vi "StartProcesses.vi"(8 "error in (no error)":errorcluster, 11 "SMO":refnum<class "SMO.lvclass">) -> (0 "error out":errorcluster, 3 "SMO out":refnum<class "SMO.lvclass">)   [LabVIEW 2013, in "SMO.lvclass"]
doc: "---------------------------------------------------------------\nJKI State Machine Objects™\nhttp://jki.net/state-machine-objects/\nCopyright (C) 2005-2015, JKI <info@jki.net>\nALL RIGHTS RESERVED"
uses:
  SMO.lvclass
panel:
  # "For instructions on how to use the JKI State Machine Objects, examples and video tutorials, visit:\nhttp://jki.net/state-machine-objects/\n\nJKI State Machine Objects™\nhttp://jki.net/state-machine-objects/\nCopyright (C) 2005-2015, JKI <info@jki.net>\nALL RIGHTS RESERVED"
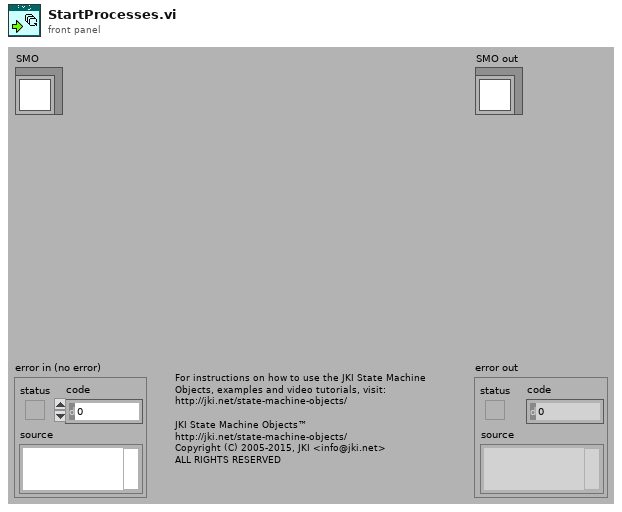
[diagram p1: front panel]
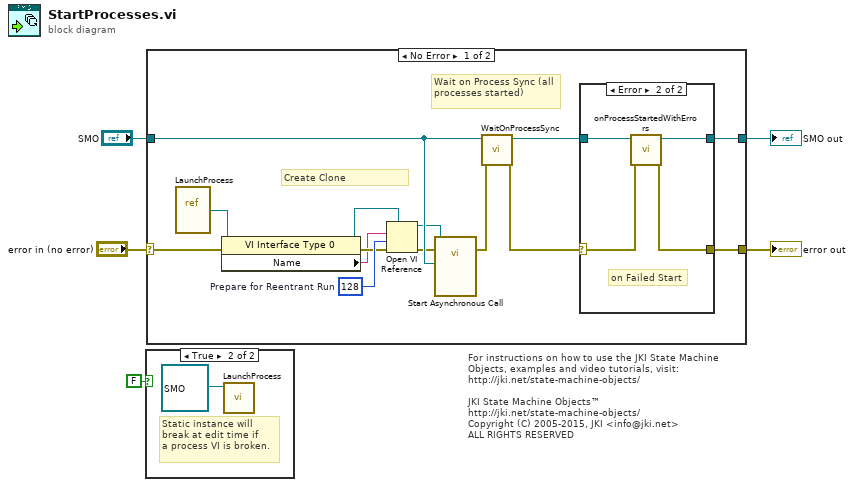
[diagram p0: block diagram]
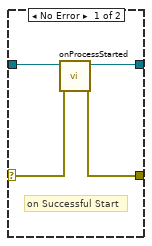
[diagram p3: hidden frame]
diagram:
  # "For instructions on how to use the JKI State Machine Objects, examples and video tutorials, visit:\nhttp://jki.net/state-machine-objects/\n\nJKI State Machine Objects™\nhttp://jki.net/state-machine-objects/\nCopyright (C) 2005-2015, JKI <info@jki.net>\nALL RIGHTS RESERVED"
  n1 = case shown="True" FALSE {
    frame False {
    }
    frame True {
      # "Static instance will\nbreak at edit time if\na process VI is broken."
      n2 = call "LaunchProcess.vi"("SMO Reference"=refnum<class "SMO.lvclass"> refnum ("JKI SMO.lvclass")) -> ()  [unwired: 11 in]
    }
  }
  n3 = case shown="No Error" "error in (no error)" {
    selector: "error in (no error)" -> [w20 w30]
    tunnel: [w17 w30] -> w2
    tunnel: "SMO" -> [w14 w29]
    tunnel: [w15 w29] -> w3
    frame No Error {
      w13 = 128  # Prepare for Reentrant Run
      # "Create Clone"
      # "Wait on Process Sync (all processes started)"
      n4 = vi-ref "LaunchProcess.vi"() -> (w9:refnum<vi>)
      n5 = property class="VI Interface Type 0"(reference=w9, error in=w20) -> (reference out=w10:refnum<vi>, error out=w12:errorcluster, "Name"=w11:string)
      n6 = Open VI Reference(type specifier VI Refnum (for type only)=w10, vi path=w11, options=w13, error in (no error)=w12) -> (vi reference=w7:refnum<vi>, error out=w8:errorcluster)  [unwired: 1 in, 1 out]
      n7 = call-by-ref "Start Asynchronous Call"(reference=w7, error in=w8, "SMO Reference"=w14) -> (error out=w19:errorcluster)  [unwired: 11 in, 1 out]
      n8 = call "WaitOnProcessSync.vi"("error in (no error)"=w19, "SMO"=w14) -> ("error out"=w16:errorcluster, "SMO out"=w18:refnum<class "SMO.lvclass">)  [unwired: 8 in]
      n9 = case shown="Error" w16 {
        selector: w16 -> [w22 w26]
        tunnel: w18 -> [w24 w28]
        tunnel: [w21 w25] -> w17
        tunnel: [w23 w27] -> w15
        frame No Error {
          # "on Successful Start"
          n10 = call-dynamic "onProcessStarted.vi"("error in (no error)"=w22, "SMO"=w24) -> ("error out"=w21:errorcluster, "SMO out"=w23:refnum<class "SMO.lvclass">)  [unwired: 8 in]
        }
        frame Error {
          # "on Failed Start"
          n11 = call-dynamic "onProcessStartedWithErrors.vi"("error in (no error)"=w26, "SMO"=w28) -> ("error out"=w25:errorcluster, "SMO out"=w27:refnum<class "SMO.lvclass">)  [unwired: 8 in]
        }
      }
    }
    frame Error {
    }
  }
  "error out" <- w2
  "SMO out" <- w3
